vi "Assert Expected Value Matches.vi"(8 "error in (no error)":errorcluster, 9 "Expected Value":u8, 10 "TestCase in":refnum<class "TestCase.lvclass">, 11 "Loopback in":refnum<class "Loopback.lvclass">) -> (0 "error out":errorcluster, 2 "TestCase out":refnum<class "TestCase.lvclass">, 3 "Loopback out":refnum<class "Loopback.lvclass">)   [LabVIEW 2020, in "Loopback.lvclass"]
uses:
  Loopback.lvclass
  <vilib>/addons/_JKI Toolkits/VI Tester/TestCase.llb/TestCase.lvclass
  Loopback.lvclass/Loopback.ctl
  <vilib>/Utility/error.llb/Error Cluster From Error Code.vi
  <vilib>/rvi/errors/niLvFpgaAdjustHostInterfaceError.vi
  <vilib>/rvi/interface/nirviReadWriteControl/nirviReadWriteControl.xnode
  NiFpgaLv.dll
  <vilib>/rvi/interface/Simulation/niFpgaSimulationCallBeginRW.vi
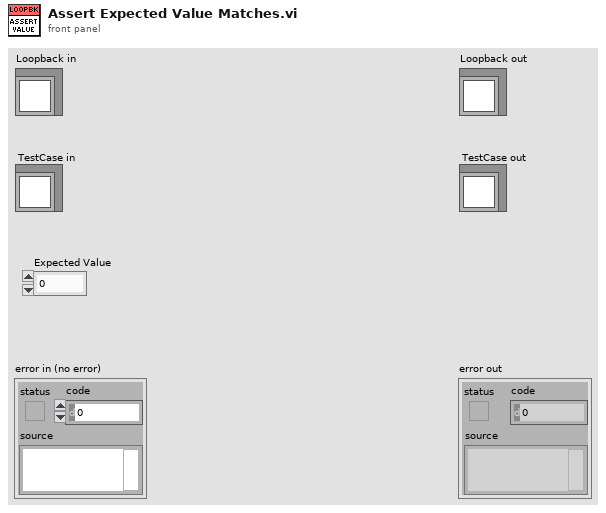
[diagram p1: front panel]
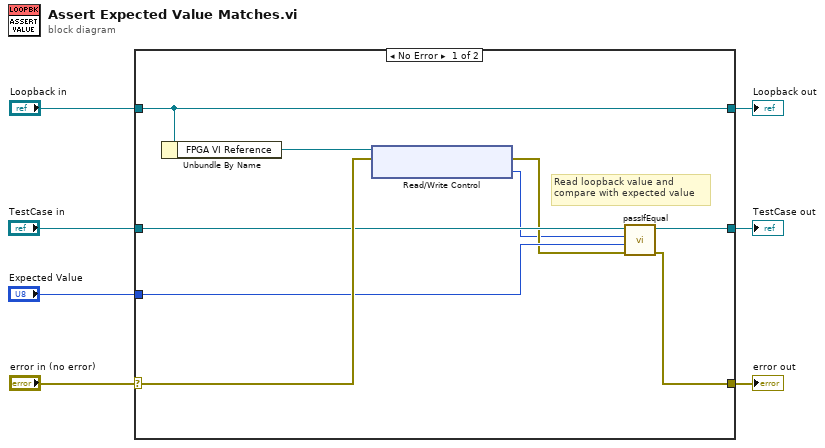
[diagram p0: block diagram]
diagram:
  n1 = case shown="No Error" "error in (no error)" {
    selector: "error in (no error)" -> [w16 w19]
    tunnel: [w9 w19] -> w6
    tunnel: [w15 w18] -> w4
    tunnel: "Loopback in" -> [w15 w18]
    tunnel: [w13 w17] -> w3
    tunnel: "TestCase in" -> [w12 w17]
    tunnel: "Expected Value" -> [w11 _]
    frame No Error {
      # "Read loopback value and\ncompare with expected value"
      n2 = Unbundle By Name(w15) -> ("FPGA VI Reference"=w14:refnum<k20>)
      n3 = xnode "Read/Write Control"("FPGA VI Reference In"=w14, "error in"=w16) -> ("error out"=w10:errorcluster, "Connector0/DIOPORT2"=w8:u8)  [unwired: 1 out]
      n4 = call-dynamic "passIfEqual.vi"("error in (no error)"=w10, "y"=w11, "x"=w8, "TestCase in"=w12) -> ("error out"=w9:errorcluster, "TestCase out"=w13:refnum<class "TestCase.lvclass">)  [unwired: 6 in]
    }
    frame Error {
    }
  }
  "error out" <- w6
  "Loopback out" <- w4
  "TestCase out" <- w3
